vi "Audio Loopback Example.vi"() -> ()   [LabVIEW 2020]
doc: "Simple example of audio device capture, saving the acquired data to a WAV file."
uses:
  Controls/Audio Device Config.ctl
  Controls/Audio Device Format.ctl
  Controls/Audio File Info.ctl
  Controls/WAV Codec Specific Info.ctl
  Controls/WAV Container Format.ctl
  Controls/WAV Data Format.ctl
  Controls/Backends.ctl
  Controls/Audio Device Info.ctl
  Controls/Audio Device Type.ctl
  Controls/Audio Device Native Data Format.ctl
  d37775a1-27ef-4781-ba3e-b38a0bb78134.vi
  7b5afa26-ffc7-4768-ab84-ffe08a27723a.vi
  12cef21b-ac69-4f16-915d-a38cc65718a6.vi
  Private/Debug Path.vi
  Private/Result To Error.vi
  d37775a1-27ef-4781-ba3e-b38a0bb78134.vi/6b901882-6109-4f44-aca5-48e1525e5248.vi
  d37775a1-27ef-4781-ba3e-b38a0bb78134.vi/06c0137a-63d3-4e30-982f-115d83a1188c.vi
  Audio Devices/Get Audio Device Configuration.vi
  Private/Audio Device Refnum To Value.vi
  7b5afa26-ffc7-4768-ab84-ffe08a27723a.vi/fba40667-3e21-44fa-934c-95909d78721c.vi
  Private/Audio File Refnum To Value.vi
  d37775a1-27ef-4781-ba3e-b38a0bb78134.vi/06c0137a-63d3-4e30-982f-115d83a1188c.vi/4b7b629c-2e91-4160-9820-a26af8f6e677.vi
  7b5afa26-ffc7-4768-ab84-ffe08a27723a.vi/fba40667-3e21-44fa-934c-95909d78721c.vi/4b7b629c-2e91-4160-9820-a26af8f6e677.vi
  Audio Files/Polymorphic VIs/Open Audio File Write (WAV).vi
  <vilib>/Utility/Data Type/Get Numeric Information.vi
  <vilib>/Utility/file.llb/Application Directory.vi
  <vilib>/Utility/error.llb/Error Cluster From Error Code.vi
  G-Audio.lvlib
panel:
  out "error out":errorcluster
  in  "Stop":bool
  out "Waveform":waveform(i16)[](graph)
  # "Instructions:\n1. Run the VI.\n2. Choose a WAV file location to save the captured audio data to.\n3. The VI will begin audio capture and display the data in the waveform graph.\n4. Press Stop to finish audio capture, and save the WAV fle.\n5. Listen to the recorded WAV with Audio Device Playback Example (G-Audio).vi."
  # "G"
  # "-Audio"
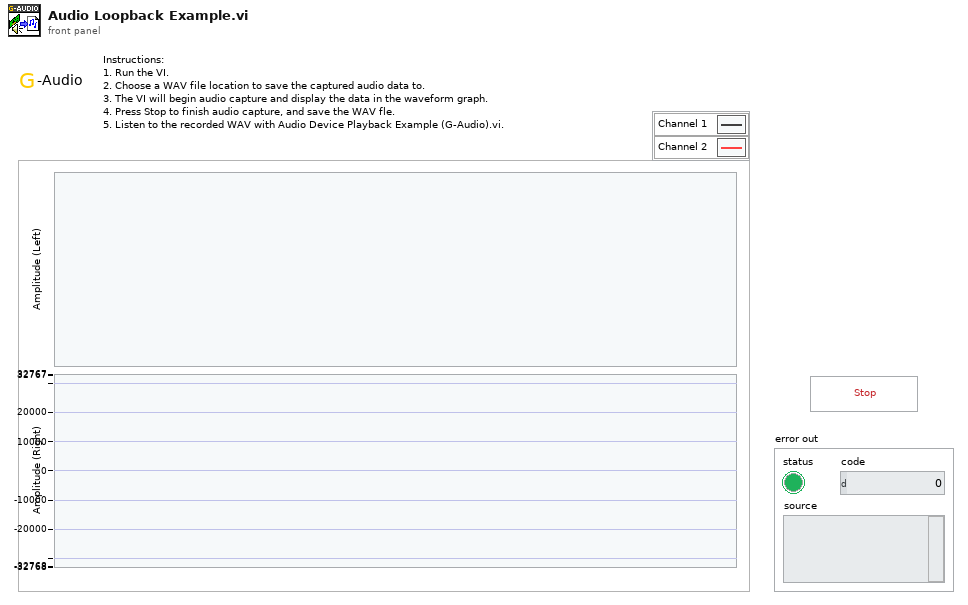
[diagram p1: front panel]
types:
  T1 = typedef "G-Audio.lvlib/Audio Device Type.ctl" = enum16{"(None)", "Playback", "Capture", "Duplex", "Loopback"}
  T2 = typedef "G-Audio.lvlib/Audio Device Info.ctl" = cluster{"Name":string, "ID":u8[], "Device Type":T1, "Default":bool, "Native Data Formats":T3[]}
  T3 = typedef "G-Audio.lvlib/Audio Device Native Data Format.ctl" = cluster{"Format":T4, "Channels":u32, "Sample Rate (Hz)":u32, "Exclusive Mode":bool}
  T4 = typedef "G-Audio.lvlib/Audio Device Format.ctl" = enum16{"Native", "U8", "I16", "I32", "SGL"}
  T5 = typedef "G-Audio.lvlib/Backends.ctl" = enum16{"WASAPI", "DirectSound", "WinMM", "Core Audio", "sndio", "audio(4)", "OSS", "PulseAudio", "ALSA", "JACK", "AAudio", "OpenSL|ES", "Web Audio", "Custom", "Null", "Default"}
  T6 = typedef "G-Audio.lvlib/WAV Codec Specific Info.ctl" = cluster{"Container Format":T7, "Data Format":T8}
  T7 = typedef "G-Audio.lvlib/WAV Container Format.ctl" = enum32{"RIFF", "Wave64"}
  T8 = typedef "G-Audio.lvlib/WAV Data Format.ctl" = u32
  T9 = typedef "G-Audio.lvlib/Audio File Info.ctl" = cluster{"Sample Rate (Hz)":u32, "Channels":u32, "Bit Depth":u32}
  T10 = typedef "G-Audio.lvlib/Audio Device Config.ctl" = cluster{"Sample Rate (Hz)":u32, "Channels":u32, "Format":T4}
  T11 = typedef "G-Audio.lvlib/Audio File Refnum.ctl" = refnum<file>
  T12 = typedef "G-Audio.lvlib/Audio Device Refnum.ctl" = refnum<file>
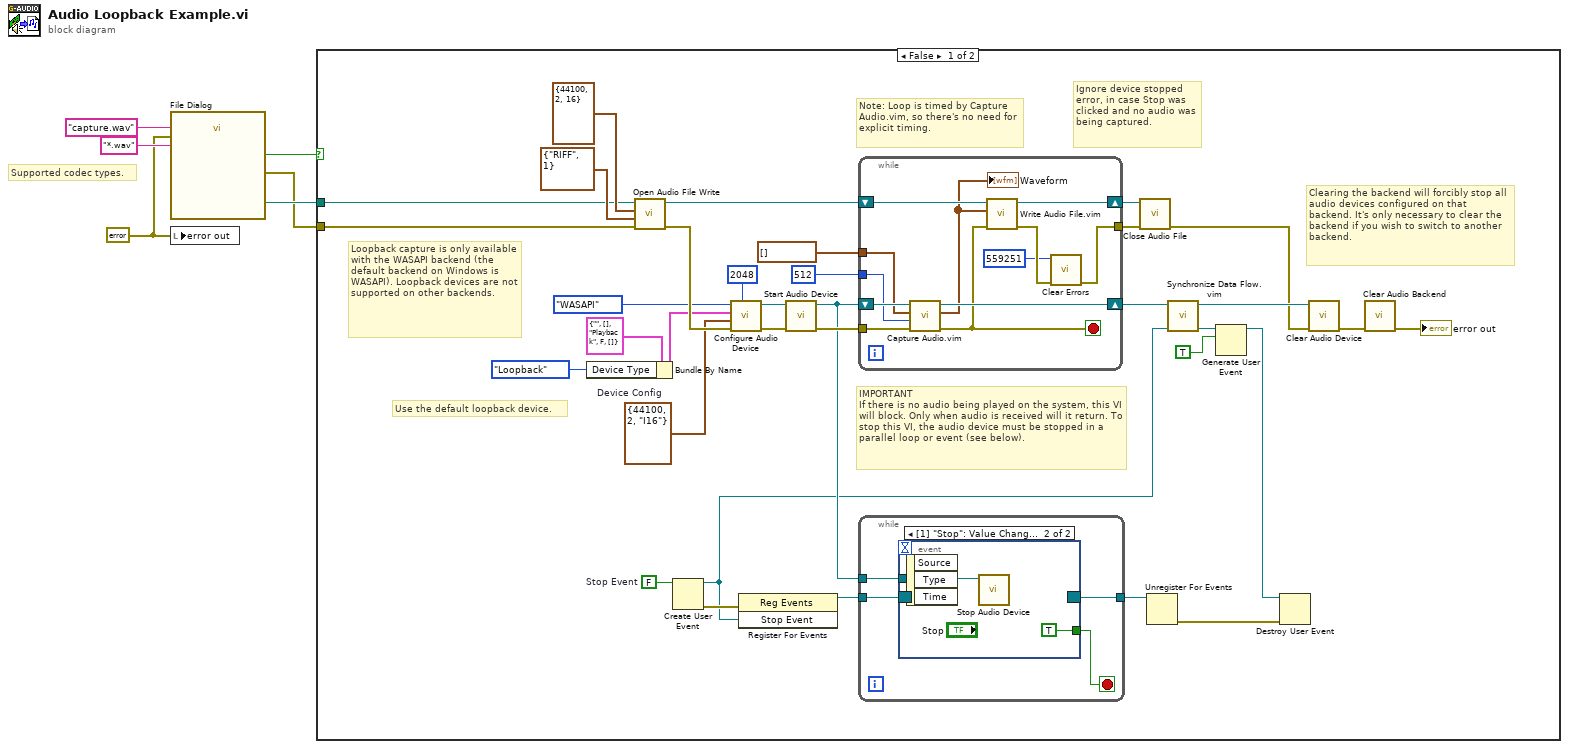
[diagram p0: block diagram]
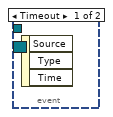
[diagram p2: hidden frame]
diagram:
  w2 = errorcluster {"status"=FALSE, "code"=0, "source"=""} ("error out")
  # "Supported codec types."
  n1 = call "File Dialog"("default name"="capture.wav", "error in"=w2, "pattern (all files)"="*.wav") -> ("selected path"=w5:path, "cancelled"=w4:bool, "error out"=w3:errorcluster)  [unwired: 9 in, 1 out]
  n2 = local write "error out"(w2) -> ()
  n3 = case shown="False" w4 {
    tunnel: w5 -> [w25 _]
    tunnel: w3 -> [w28 _]
    frame False {
      w20 = FALSE  # Stop Event
      w30 = T10 {"Sample Rate (Hz)"=44100, "Channels"=2, "Format"=enum."I16"}  # Device Config
      # "Use the default loopback device."
      # "Ignore device stopped error, in case Stop was clicked and no audio was being captured."
      # "IMPORTANT\nIf there is no audio being played on the system, this VI will block. Only when audio is received will it return. To stop this VI, the audio device must be stopped in a parallel loop or event (see below)."
      # "Loopback capture is only available with the WASAPI backend (the default backend on Windows is WASAPI). Loopback devices are not supported on other backends."
      # "Clearing the backend will forcibly stop all audio devices configured on that backend. It's only necessary to clear the backend if you wish to switch to another backend."
      # "Note: Loop is timed by Capture Audio.vim, so there's no need for explicit timing."
      n4 = Bundle By Name(cluster=T2 {"Name"="", "ID"=[], "Device Type"=enum."Playback", "Default"=FALSE, "Native Data Formats"=[]} ("Audio Device"), "Device Type"=Audio_Device_Type."Loopback") -> (w7:T2)
      n5 = call-poly "Open Audio File Write.vi"("error in (no error)"=w28, "Codec Specific Info"=T6 {"Container Format"=enum."RIFF", "Data Format"=1}, "Audio File Info"=T9 {"Sample Rate (Hz)"=44100, "Channels"=2, "Bit Depth"=16}, "Path"=w25) -> ("error out"=w34:errorcluster, "Audio File Refnum"=w36:T11)  [unwired: 6 in]
      n6 = Create User Event(user event datatype=w20) -> (user event=w14:refnum<user-event>, error out=w22:errorcluster)  [unwired: 1 in]
      n7 = call "Configure Audio Device.vi"("Buffer Size (4096)"=2048 ("number of samples/ch"), "error in (no error)"=w34, "Device Config"=w30, "Audio Device"=w7, "Backend (Default)"=Backends."WASAPI") -> ("error out"=w33:errorcluster, "Audio Device Refnum"=w32:T12)  [unwired: 3 in, 2 out]
      n8 = register-events(error in=w22, w14) -> (reference out=w21:refnum<event-registration>)  [unwired: 1 in, 1 out]
      n9 = call "Start Audio Device.vi"("error in (no error)"=w33, "Audio Device Refnum In"=w32) -> ("error out"=w38:errorcluster, "Audio Device Refnum Out"=w23:T12)  [unwired: 8 in]
      n10 = while {
        shift-right: [w56] -> w40
        shift-left: w36 -> [w58]
        shift-right: [w55] -> w16
        shift-left: w23 -> [w57]
        tunnel: w38 -> [w52]
        tunnel: [w50] -> w39
        tunnel: 512 ("number of samples/ch") -> [w54]
        tunnel: waveform(i16)[] [] -> [w53]
        stop <- w47 stop-if-true
        n11 = call "Capture Audio.vim"("error in (no error)"=w52, "Samples To Read"=w54, "Data Format"=w53, "Audio Device Refnum In"=w57) -> ("error out"=w47:errorcluster, "Audio Data"=w48:waveform(i16)[], "Audio Device Refnum Out"=w55:T12)  [unwired: 5 in]
        "Waveform" <- w48
        n12 = call "Write Audio File.vim"("error in (no error)"=w47, "Audio Data"=w48, "Audio File Refnum In"=w58) -> ("error out"=w51:errorcluster, "Audio File Refnum Out"=w56:T11)  [unwired: 7 in]
        n13 = call <vilib>:"Clear Errors.vi"("error in (no error)"=w51, "specific error code to clear (0: all)"=559251) -> ("error out"=w50:errorcluster)  [unwired: 4 in, 1 out]
      }
      n14 = while {
        tunnel: w23 -> [w44]
        tunnel: w21 -> [w42]
        tunnel: [w41] -> w18
        stop <- w43 stop-if-true
        n15 = event shown="[1] \"Stop\": Value Change;  <Stop Event>: User Event" {
          selector: w42 -> [_ _]
          dyn-events: [_ _] -> w41
          timeout: _ -> [_ _]
          tunnel: w44 -> [_ w46]
          tunnel: [_ TRUE] -> w43
          event Timeout {
            n16 = event-data() -> ()  [unwired: 1 in, 3 out]
          }
          event "Stop": Value Change; User Event {
            n17 = event-data() -> ()  [unwired: 1 in, 3 out]
            n18 = call "Stop Audio Device.vi"("Audio Device Refnum In"=w46) -> ()  [unwired: 9 in, 2 out]
          }
        }
      }
      n19 = call "Close Audio File.vi"("error in (no error)"=w39, "Audio File Refnum In"=w40) -> ("error out"=w12:errorcluster)  [unwired: 9 in]
      n20 = Unregister For Events(event registration refnum=w18) -> (error out=w17:errorcluster)  [unwired: 1 in]
      n21 = call "Synchronize Data Flow.vim"("input 4"=w14, "input 1"=w16) -> ("output 4"=w13:refnum<user-event>, "output 1"=w15:T12)  [unwired: 2 in, 2 out]
      n22 = Generate User Event(user event=w13, event data cluster=TRUE ("event data")) -> (user event out=w11:refnum<user-event>)  [unwired: 2 in, 1 out]
      n23 = Destroy User Event(user event=w11, error in=w17) -> ()  [unwired: 1 out]
      n24 = call "Clear Audio Device.vi"("error in (no error)"=w12, "Audio Device Refnum In"=w15) -> ("error out"=w37:errorcluster)  [unwired: 9 in]
      n25 = call "Clear Audio Backend.vi"("error in (no error)"=w37) -> ("error out"=→"error out":errorcluster)  [unwired: 10 in]
    }
    frame True {
    }
  }
